vi "Write_Variable.vi"(2 "Value":string="10", 3 "Variable name":string="CDTIME", 4 "Service":string="ROBCOMM") -> ()   [LabVIEW 2012]
panel:
  out "Command":string="VARIABLE"
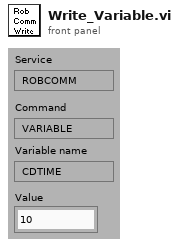
[diagram p1: front panel]
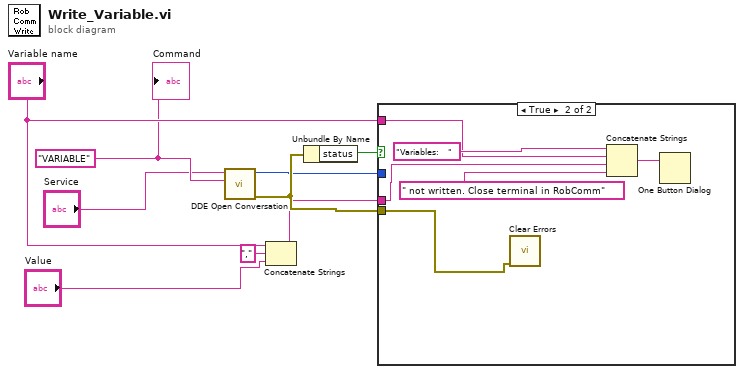
[diagram p0: block diagram]
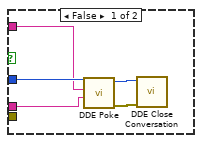
[diagram p2: hidden frame]
diagram:
  w2 = "VARIABLE" ("topic")
  n1 = call <vilib>:"DDE Open Conversation.vi"("topic"=w2, "service"="Service") -> ("error out"=w9:errorcluster, "conversation refnum"=w3:u32)  [unwired: 6 in]
  n2 = Concatenate Strings("Variable name", "," ("string"), "Value") -> (w7:string)
  n3 = Unbundle By Name(w9) -> ("status"=w8:bool)
  n4 = case shown="True" w8 {
    tunnel: w3 -> [w14 _]
    tunnel: "Variable name" -> [w11 w19]
    tunnel: w7 -> [w10 w16]
    tunnel: w9 -> [_ w15]
    frame False {
      n5 = call <vilib>:"DDE Poke.vi"("data"=w10, "item"=w11, "conversation refnum in"=w14) -> ("error out"=w12:errorcluster, "conversation refnum out"=w13:u32)  [unwired: 5 in]
      n6 = call <vilib>:"DDE Close Conversation.vi"("error in (no error)"=w12, "conversation refnum"=w13) -> ()  [unwired: 7 in, 1 out]
    }
    frame True {
      n7 = call <vilib>:"Clear Errors.vi"("error in (no error)"=w15) -> ()  [unwired: 6 in, 1 out]
      n8 = Concatenate Strings("Variables:   " ("string"), w19, w16, " not written. Close terminal in RobComm" ("string")) -> (w18:string)
      n9 = One Button Dialog(message=w18) -> ()  [unwired: 1 in, 1 out]
    }
  }
  "Command" <- w2
